vi "CenterFrontPanelTest.vi"   [LabVIEW 2018]
uses:
  <vilib>/Utility/miscctls.llb/LVRectTypeDef.ctl
types:
  T1 = typedef "LVRectTypeDef.ctl" = cluster{"Left":i16, "Top":i16, "Right":i16, "Bottom":i16}
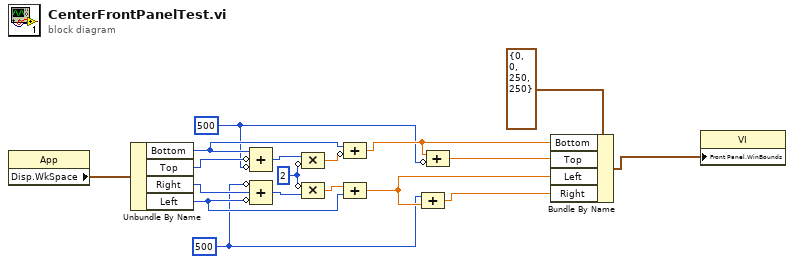
[diagram p0: block diagram]
diagram:
  w2 = i16 500 ("Right")
  w13 = i16 2 ("Right")
  w1 = i16 500 ("Right")
  n1 = property class="App"() -> ("Disp.WkSpace"=w18:T1)  [unwired: 2 in, 2 out]
  n2 = Unbundle By Name(w18) -> ("Bottom"=w10:i16, "Top"=w16:i16, "Right"=w17:i16, "Left"=w7:i16)
  n3 = Compound Arithmetic op=ADD(w10, invert w16, invert w1) -> (w14:i16)
  n4 = Compound Arithmetic op=ADD(invert w2, w17, invert w7) -> (w15:i16)
  n5 = Compound Arithmetic op=MULTIPLY(w14, invert w13) -> (w9:dbl)
  n6 = Compound Arithmetic op=MULTIPLY(invert w13, w15) -> (w8:dbl)
  n7 = Compound Arithmetic op=ADD(w10, invert w9) -> (w5:dbl)
  n8 = Compound Arithmetic op=ADD(w8, w7) -> (w6:dbl)
  n9 = Compound Arithmetic op=ADD(w2, w6) -> (w3:dbl)
  n10 = Compound Arithmetic op=ADD(w5, invert w1) -> (w4:dbl)
  n11 = Bundle By Name(cluster=T1 {"Left"=0, "Top"=0, "Right"=250, "Bottom"=250} ("Front Panel Window:Window Bounds"), "Bottom"=w5, "Top"=w4, "Left"=w6, "Right"=w3) -> (w11:T1)
  n12 = property class="VI"("Front Panel.WinBounds"=w11) -> ()  [unwired: 2 in, 2 out]
